vi "Stop.vi"   [LabVIEW 2012]
uses:
  Globals.vi
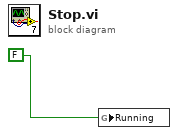
[diagram p0: block diagram]
diagram:
  n1 = global write "Globals.vi" "Running"(FALSE) -> ()
